vi "Convert R to T - DBL Array.vi"(8 "error in":errorcluster, 9 "R (kO)":dbl[](array[numeric])=[3.893, 10.0, 29.49], 10 "Tref (C)":dbl[](array[numeric])=[50.0, 25.0, 0.0], 11 "R":dbl[](array[numeric]) caption="R (kOhm)") -> (0 "error out":errorcluster, 3 "T":dbl[](array[numeric]) caption="T (degC)")   [LabVIEW 2015, in "Temperature.lvlib"]
doc: "Converts an array of thermistor resistance in kOhms to an array of temperature a temperature in degrees Celsius"
uses:
  Temperature.lvlib
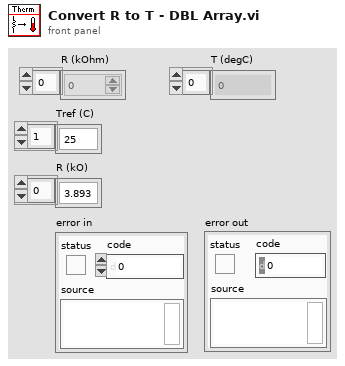
[diagram p1: front panel]
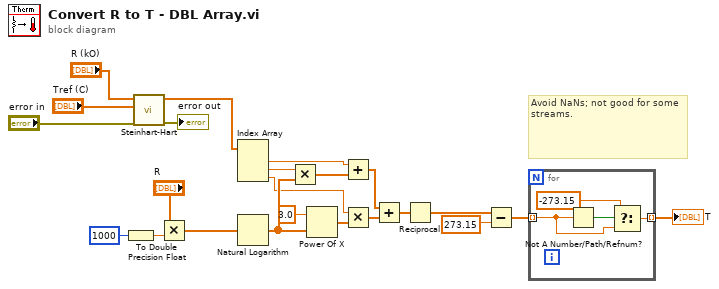
[diagram p0: block diagram]
diagram:
  # "Avoid NaNs; not good for some streams."
  n1 = To Double Precision Float(number=1000) -> (double precision float=w3:dbl)
  n2 = call "Steinhart-Hart.vi"("error in"="error in", "Tref (C)"="Tref (C)", "R (kO)"="R (kO)") -> ("error out"=→"error out":errorcluster, "Coefficients"=w23:dbl[])  [unwired: 7 in]
  n3 = Multiply(x="R", y=w3) -> (x*y=w9:dbl[])
  n4 = Index Array(array=w23) -> (element #1=w22:dbl, element #2=w20:dbl, element #3=w17:dbl)  [unwired: 3 in]
  n5 = Natural Logarithm(1:w9) -> (0:w19:dbl[])
  n6 = Multiply(x=w20, y=w19) -> (x*y=w18:dbl[])
  n7 = Power Of X(1:w19, 2:3.0 ("y")) -> (0:w16:dbl[])
  n8 = Add(x=w22, y=w18) -> (x+y=w14:dbl[])
  n9 = Multiply(x=w17, y=w16) -> (x*y=w15:dbl[])
  n10 = Add(x=w14, y=w15) -> (x+y=w13:dbl[])
  n11 = Reciprocal(x=w13) -> (1/x=w12:dbl[])
  n12 = Subtract(x=w12, y=273.15) -> (x-y=w2:dbl[])
  n13 = for {
    tunnel: w2 -> [w25] mode=indexing
    tunnel: [w24] -> w1 mode=indexing
    n14 = Not A Number/Path/Refnum?(number/path/refnum=w25) -> (NaN/Path/Refnum?=w27:bool)
    n15 = Select(t=-273.15, s=w27, f=w25) -> (s? t:f=w24:dbl)
  }
  "T" <- w1
